vi "Collapse All.vi"(8 "error in (no error)":errorcluster, 11 "MenuButton Event Handler in":refnum<class "MenuButton Event Handler.lvclass">) -> (0 "error out":errorcluster, 3 "MenuButton Event Handler out":refnum<class "MenuButton Event Handler.lvclass">)   [LabVIEW 2017, in "MenuButtons.lvlib" / "MenuButton Event Handler.lvclass"]
uses:
  MenuButton Event Handler.lvclass
  MenuButton Event Handler.lvclass/MenuButton Event Handler.ctl
  MenuButton/MenuButton.lvclass/MenuButton.ctl
  MenuButton/MenuButton.lvclass
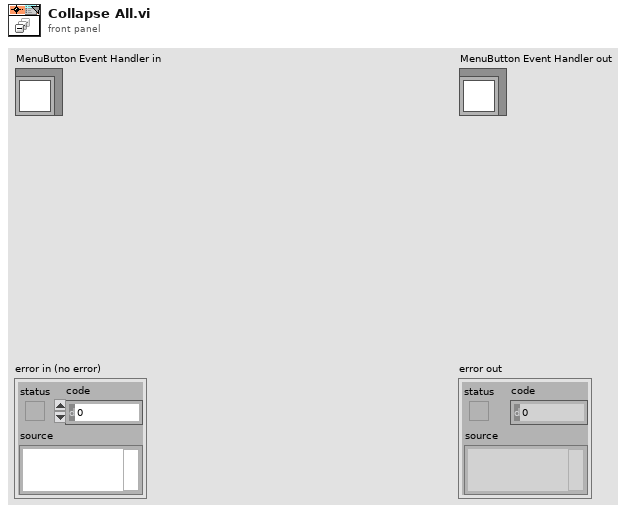
[diagram p1: front panel]
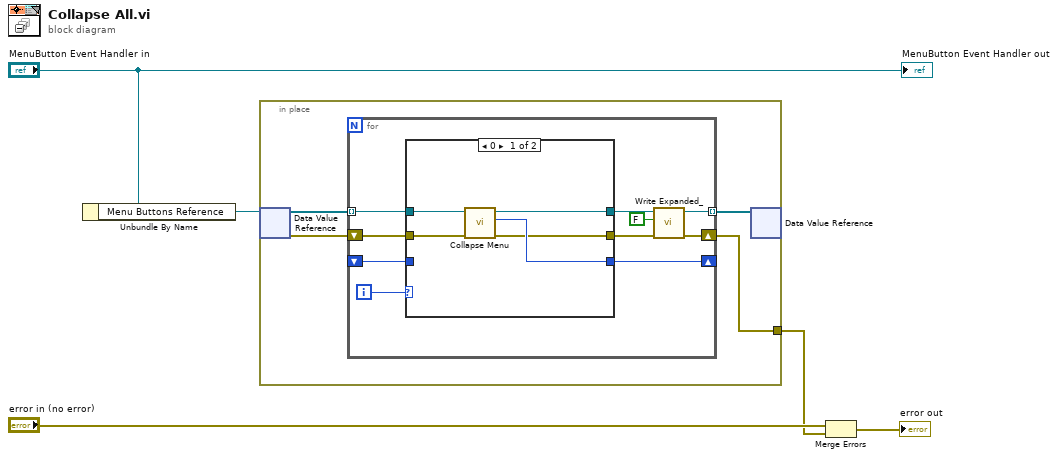
[diagram p0: block diagram]
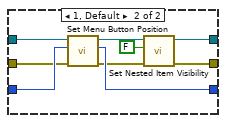
[diagram p2: hidden frame]
diagram:
  n1 = Unbundle By Name("MenuButton Event Handler in") -> ("Menu Buttons Reference"=w3:refnum<data-value>)
  n2 = in-place {
    in-place-border: [w6] -> w1
    n3 = in-place-dvr #1(w3) -> (w9:refnum<class "MenuButton.lvclass">[], w7:errorcluster)
    n4 = for {
      tunnel: w9 -> [w19] mode=indexing
      tunnel: [w14] -> w8 mode=indexing
      shift-right: [w17] -> _
      shift-left: _ -> [w16]
      shift-right: [w10] -> w6
      shift-left: w7 -> [w12]
      i -> [w18]
      n5 = case shown="0" w18 {
        tunnel: w19 -> [w24 w32]
        tunnel: [w23 w31] -> w15
        tunnel: [w22 w29] -> w17
        tunnel: w16 -> [_ w30]
        tunnel: w12 -> [w21 w26]
        tunnel: [w20 w25] -> w11
        frame 0 {
          n6 = call "Collapse Menu.vi"("error in (no error)"=w21, "MenuButton in"=w24) -> ("error out"=w20:errorcluster, "Menu Bottom Position"=w22:u32, "MenuButton out"=w23:refnum<class "MenuButton.lvclass">)  [unwired: 7 in]
        }
        frame 1, Default {
          n7 = call "Set Menu Button Position.vi"("error in (no error)"=w26, "Top Position"=w30, "MenuButton in"=w32) -> ("error out"=w27:errorcluster, "Bottom Postion"=w29:u32, "MenuButton out"=w33:refnum<class "MenuButton.lvclass">)  [unwired: 6 in]
          n8 = call "Set Nested Item Visibility.vi"("error in (no error)"=w27, "Visible?"=FALSE, "MenuButton in"=w33) -> ("error out"=w25:errorcluster, "MenuButton out"=w31:refnum<class "MenuButton.lvclass">)  [unwired: 7 in]
        }
      }
      n9 = call "Write Expanded_.vi"("error in (no error)"=w11, "Expanded?"=FALSE, "MenuButton in"=w15) -> ("error out"=w10:errorcluster, "MenuButton out"=w14:refnum<class "MenuButton.lvclass">)  [unwired: 7 in]
    }
    n10 = in-place-dvr #1(w8) -> ()  [unwired: 2 out]
  }
  n11 = Merge Errors("error in (no error)", w1) -> (→"error out":errorcluster)
  "MenuButton Event Handler out" <- "MenuButton Event Handler in"
